vi "test.vi"(1 "String":string, 2 "number":i32) -> (0 "concatenated string":string)   [LabVIEW 2009]
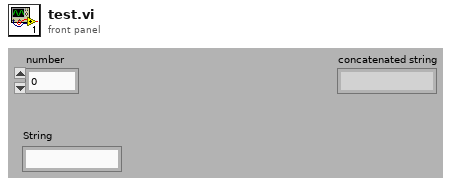
[diagram p1: front panel]
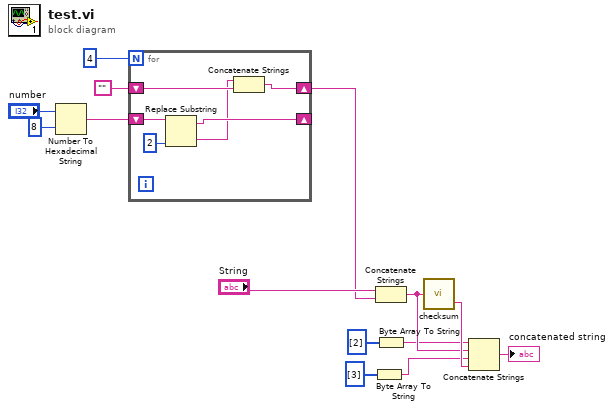
[diagram p0: block diagram]
diagram:
  n1 = Number To Hexadecimal String(1:i16 8 ("width (-)"), 2:"number") -> (0:w4:string)
  n2 = for {
    N: 4 -> [_]
    shift-right: [w17] -> _
    shift-left: w4 -> [w20]
    shift-right: [w15] -> w1
    shift-left: "" -> [w18]
    n3 = Replace Substring(2:2 ("length (len. of substring)"), 5:w20) -> (0:w16:string, 1:w17:string)  [unwired: 2 in]
    n4 = Concatenate Strings(w16, w18) -> (w15:string)
  }
  n5 = Byte Array To String(unsigned byte array=u8[] [3]) -> (string=w13:string)
  n6 = Concatenate Strings("String", w1) -> (w12:string)
  n7 = Byte Array To String(unsigned byte array=u8[] [2]) -> (string=w10:string)
  n8 = call "checksum.vi"("Data"=w12) -> ("Check Sum"=w14:string)  [unwired: 2 in, 1 out]
  n9 = Concatenate Strings(w10, w12, w13, w14) -> (→"concatenated string":string)
